vi "Send.vi"(8 "error in":errorcluster, 11 "Block Upload End Transfer in":refnum<class "Block Upload End Transfer.lvclass">) -> (0 "error out":errorcluster)   [LabVIEW 2020, in "CANopen.lvlib" / "SDO Manager.lvlib" / "Block Upload End Transfer.lvclass"]
uses:
  Block Upload End Transfer.lvclass
  HAL/Source/Interfaces/ICommunicate/ICommunicate.lvclass
  CANopen Message/CANopen Message.lvclass
  Block Upload End Transfer.lvclass/Block Upload End Transfer.ctl
  D:/git/CANopen-LabVIEW/source/SDO Manager/SDO Manager/SDO Transfer/SDO Transfer.lvclass
  D:/git/CANopen-LabVIEW/source/SDO Manager/SDO Manager/Block Upload End Transfer/Block Upload End Transfer.lvclass
  Typedefs/Function Code.ctl
  CANopen.lvlib
  SDO Transfer/SDO Transfer.lvclass
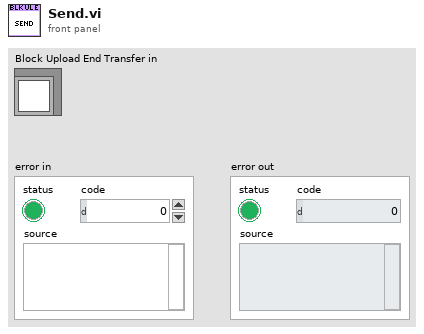
[diagram p1: front panel]
types:
  T1 = typedef "CANopen.lvlib/Function Code.ctl" = u8
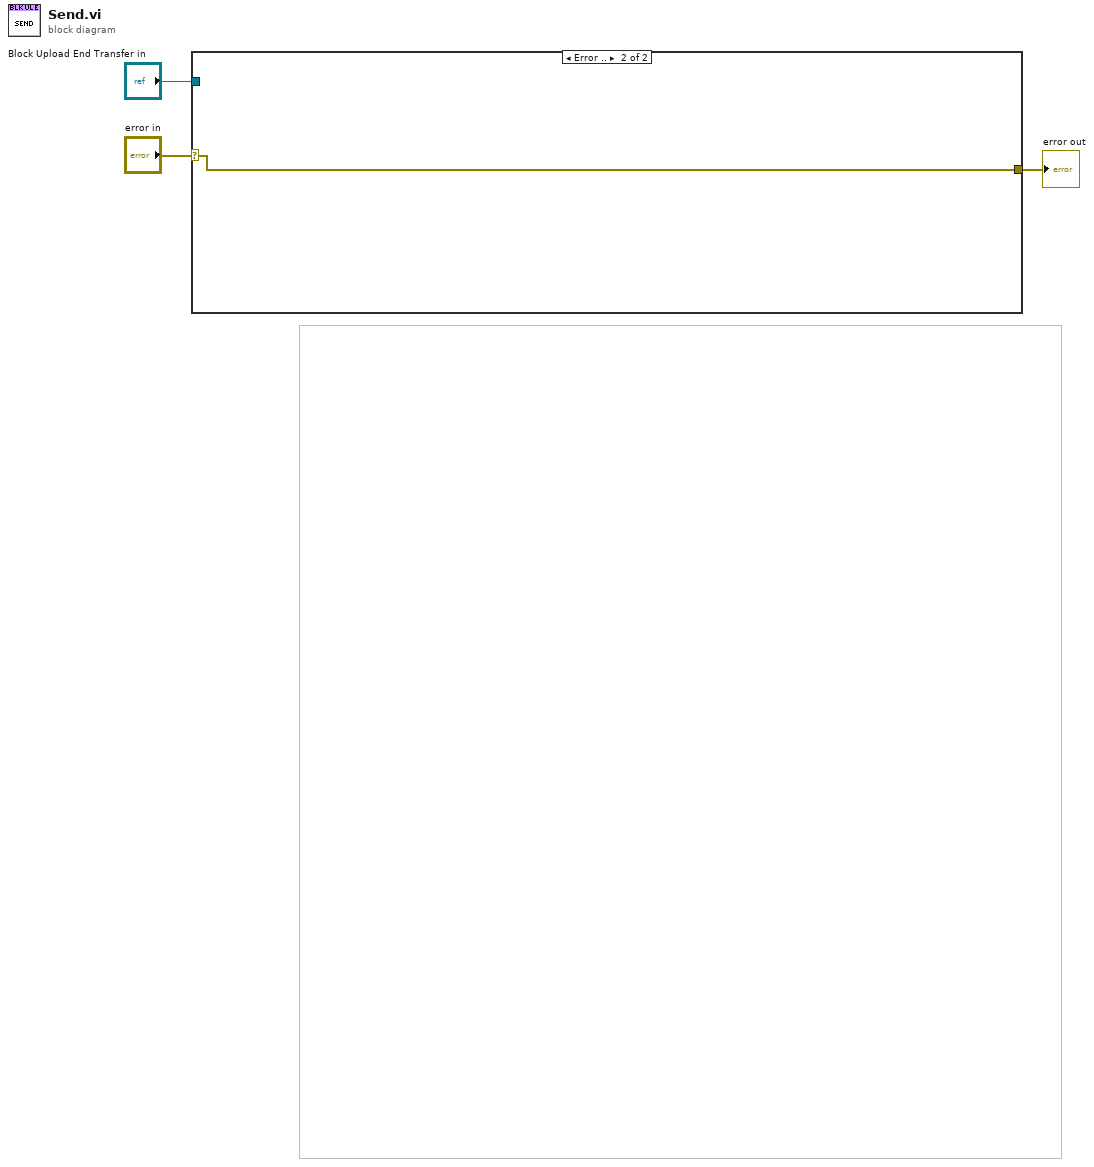
[diagram p0: block diagram]
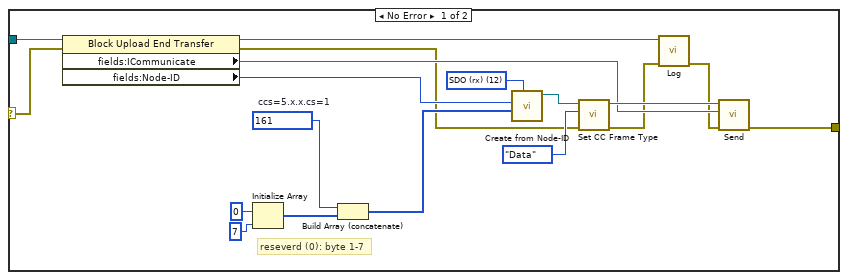
[diagram p2: hidden frame]
diagram:
  n1 = case shown="Error .." "error in" {
    selector: "error in" -> [w21 w22]
    tunnel: "Block Upload End Transfer in" -> [w20 _]
    tunnel: [w8 w22] -> w1
    frame No Error {
      w15 = T1 12 items=["NMT"=0, "EMCY/SYNC"=1, "TIME"=2, "PDO1 (tx)"=3, "PDO1 (rx)"=4, "PDO2 (tx)"=5, "PDO2 (rx)"=6, "PDO3 (tx)"=7, "PDO3 (rx)"=8, "PDO4 (tx)"=9, "PDO4 (rx)"=10, "SDO (tx)"=11, "SDO (rx)"=12, "NMT error control"=14] ("Function Code")
      w18 = u8 161  # ccs=5.x.x.cs=1
      # "reseverd (0): byte 1-7"
      n2 = property class="Block Upload End Transfer"(reference=w20, error in=w21) -> (reference out=w9:refnum<class "Block Upload End Transfer.lvclass">, error out=w7:errorcluster, "fields:ICommunicate"=w10:refnum<class "ICommunicate.lvclass">, "fields:Node-ID"=w19:u8)
      n3 = Initialize Array(u8 0, 7 ("y")) -> (w4:u8[])
      n4 = Build Array (concatenate)(w18, w4) -> (w16:u8[])
      n5 = call "Create from Node-ID.vi"("Function Code"=w15, "Data"=w16, "Node-ID"=w19) -> ("CANopen Message"=w14:refnum<class "CANopen Message.lvclass">)  [unwired: 8 in]
      n6 = call "Set CC Frame Type.vi"("error in"=w7, "CC Frame Type"=enum8{"Data", "Remote", "Error", "Overload"}."Data", "CANopen Message in"=w14) -> ("error out"=w6:errorcluster, "CANopen Message out"=w13:refnum<class "CANopen Message.lvclass">)  [unwired: 7 in]
      n7 = call "Log.vi"("error in"=w6, "SDO Transfer in"=w9) -> ("error out"=w5:errorcluster)  [unwired: 9 in]
      n8 = call "Send.vi"("error in"=w5, "ICommunicate"=w10, "CANopen Message in"=w13) -> ("error out"=w8:errorcluster)  [unwired: 7 in, 1 out]
    }
    frame Error {
    }
  }
  "error out" <- w1
